vi "main.vi"() -> ()   [LabVIEW 2018]
panel:
  in  "Byes/Double Headers":enum16{"Byes", "Double Headers"}(ring)
  in  "Type":enum16{"League (No Mix)"}(ring)
  in  "# Games per Team":enum16{""}(ring)
  in  "# Teams":enum16{""}(ring)
  # "Byes or Double Headers\nare needed when a round\ndoes not align."
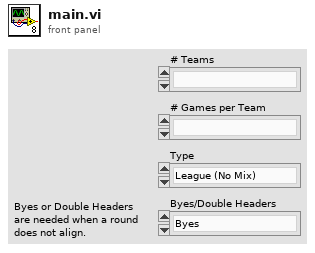
[diagram p1: front panel]
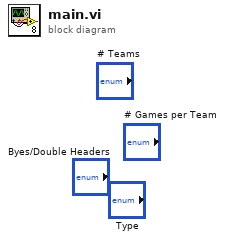
[diagram p0: block diagram]
diagram:
